vi "Lissajous XY.vi"() -> ()   [LabVIEW 2020]
panel:
  out "XY Graph":cluster{dbl[], dbl[]}[](graph)
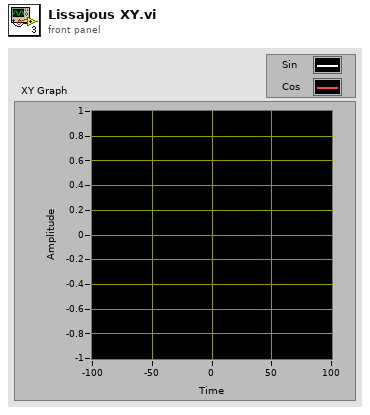
[diagram p1: front panel]
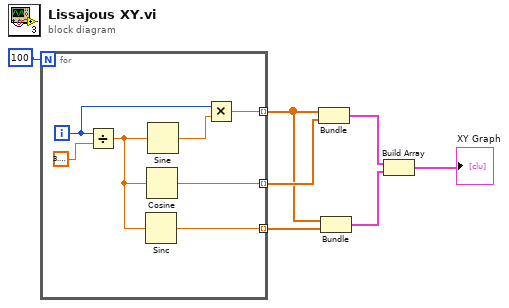
[diagram p0: block diagram]
diagram:
  n1 = for {
    N: 100 -> [_]
    tunnel: [w10] -> w4 mode=indexing
    tunnel: [w9] -> w6 mode=indexing
    tunnel: [w8] -> w5 mode=indexing
    i -> [w13]
    n2 = Divide(x=w13, y=3.141592653589793) -> (x/y=w11:dbl)
    n3 = Sinc(1:w11) -> (0:w8:dbl)
    n4 = Cosine(x=w11) -> (cos(x)=w9:dbl)
    n5 = Sine(x=w11) -> (sin(x)=w12:dbl)
    n6 = Multiply(x=w13, y=w12) -> (x*y=w10:dbl)
  }
  n7 = Bundle "Bundle"(w4, w6) -> (w3:cluster{dbl[], dbl[]})  [unwired: 1 in]
  n8 = Bundle "Bundle"(w4, w5) -> (w2:cluster{dbl[], dbl[]})  [unwired: 1 in]
  n9 = Build Array "Build Array"(w3, w2) -> (→"XY Graph":cluster{dbl[], dbl[]}[])
